vi "Serial_Write.vi"(8 "error in (no error)":errorcluster, 10 "Text to write":string, 11 "Python in":cluster{"Python":refnum<k35>, "py file":path}) -> (0 "error out":errorcluster, 3 "Python out":cluster{"Python":refnum<k35>, "py file":path})   [LabVIEW 2020]
panel:
  out "return value":string
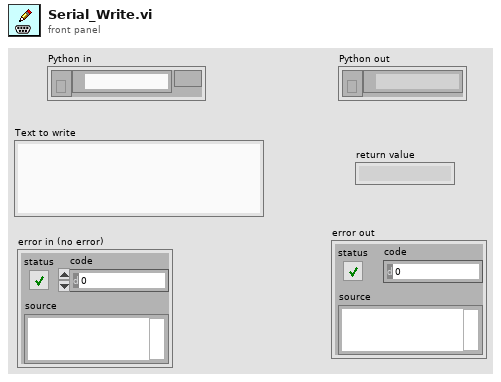
[diagram p1: front panel]
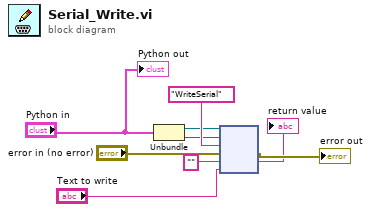
[diagram p0: block diagram]
diagram:
  n1 = Unbundle("Python in") -> ("Python"=w5:refnum<k35>, "py file"=w4:path)
  n2 = node(w5, w4, "WriteSerial" ("function name"), "error in (no error)", "" ("function name"), "Text to write") -> (→"error out":errorcluster, →"return value":string)  [unwired: 1 in, 3 out]
  "Python out" <- "Python in"
